vi "Loop.vi"() -> ()   [LabVIEW 2018]
panel:
  out "Value History":dbl(graph)
  in  "?":bool
  in  "milisecond delay":dbl(slide) scale=0.0..10.0
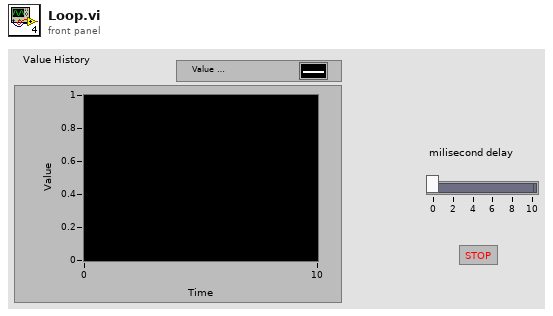
[diagram p1: front panel]
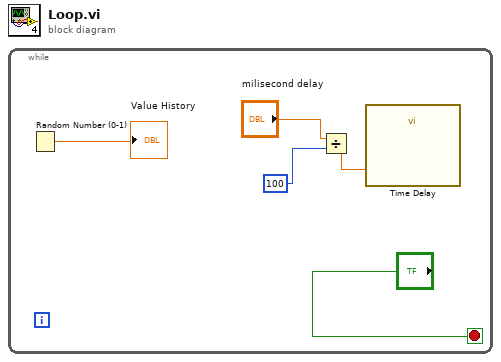
[diagram p0: block diagram]
diagram:
  n1 = while {
    stop <- "?" stop-if-true
    n2 = Random Number (0-1)() -> (number: 0 to 1=→"Value History":dbl)
    n3 = Divide(x="milisecond delay", y=100) -> (x/y=w1:dbl)
    n4 = call "Time Delay"("Delay Time (s)"=w1) -> ()  [unwired: 10 in, 1 out]
  }
